vi "PH_Countdown-Counter.contents.vi"   [LabVIEW 2014, in "PH_Countdown-Counter.lvlib"]
doc: "This class is forseen to countdown before a shot.\n\nThis class is part of the PHELIX user layer."
uses:
  PH_Countdown-Counter.lvlib
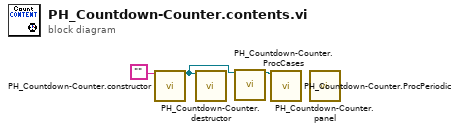
[diagram p0: block diagram]
diagram:
  n1 = call "PH_Countdown-Counter.constructor.vi"("name"="") -> ("i ref out"=w1:refnum<vi>)  [unwired: 16 in, 2 out]
  n2 = call "PH_Countdown-Counter.destructor.vi"("i ref in"=w1) -> ()  [unwired: 18 in, 1 out]
  n3 = call "PH_Countdown-Counter.ProcCases.vi"("i ref in"=w1) -> ("i ref out"=w3:refnum<vi>)  [unwired: 16 in, 2 out]
  n4 = call "PH_Countdown-Counter.ProcPeriodic.vi"("i ref in"=w3) -> ()  [unwired: 16 in, 3 out]
  n5 = call "PH_Countdown-Counter.panel.vi"() -> ()  [unwired: 1 in]
